vi "Calculate Histogram Data.vi"(7 "Switch X/Y":bool, 11 "Entries":T1[](array[typedef])) -> (3 "Histogram Data":cluster{"X":dbl, "Y":i32}[](array[cluster]))   [LabVIEW 2019, in "Muon Data Post-Processing.lvlib"]
uses:
  Muon Data Post-Processing.lvlib
  <vilib>/Utility/miscctls.llb/LVMapReplaceAction.ctl
  <vilib>/Analysis/NI_AALBase.lvlib
  <vilib>/Analysis/1siggen.llb/Ramp Pattern by Delta.vi
  File Entry.ctl
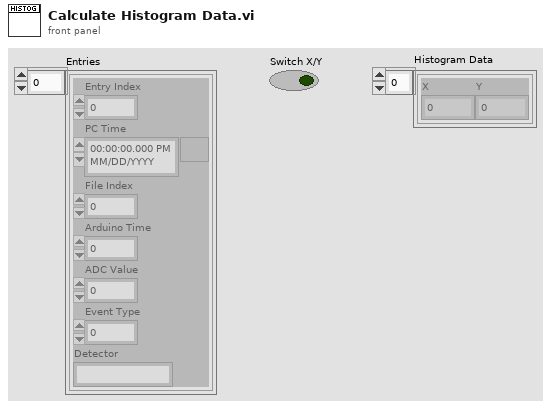
[diagram p1: front panel]
types:
  T1 = typedef "Muon Data Post-Processing.lvlib/File Entry.ctl" = cluster{"Entry Index":i32, "PC Time":timestamp, "File Index":i32, "Arduino Time":i32, "ADC Value":i32, "Event Type":i32, "Detector":string}
  T2 = typedef "LVMapReplaceAction.ctl" = enum32{"Modify Entry only if found", "Add or Modify Entry", "Delete Entry"}
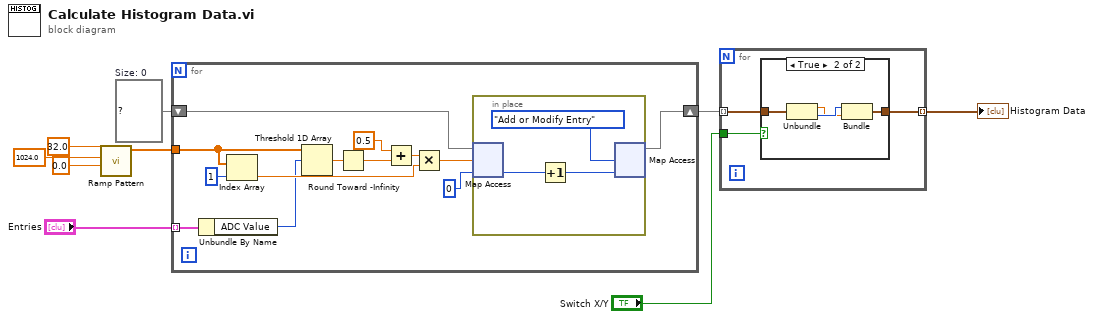
[diagram p0: block diagram]
diagram:
  w4 = map{dbl, i32} {}  # Size: 0
  n1 = call-poly <vilib>:"Ramp Pattern.vi"("start"=0.0, "end"=1024.0, "delta"=32.0) -> ("Ramp Pattern"=w5:dbl[])  [unwired: 6 in, 2 out]
  n2 = for {
    tunnel: "Entries" -> [w22] mode=indexing
    shift-right: [w12] -> w3
    shift-left: w4 -> [w11]
    tunnel: w5 -> [w10]
    n3 = Unbundle By Name(w22) -> ("ADC Value"=w15:i32)
    n4 = Index Array(array=w10, index=1) -> (element=w21:dbl)
    n5 = Threshold 1D Array(2:w15, 3:w10) -> (0:w20:dbl)  [unwired: 1 in]
    n6 = Round Toward -Infinity(1:w20) -> (0:w19:dbl)
    n7 = Add(x=0.5, y=w19) -> (x+y=w18:dbl)
    n8 = Multiply(x=w18, y=w21) -> (x*y=w14:dbl)
    n9 = in-place {
      n10 = in-place-map #1(w11, w14, 0) -> (w25:i32)  [unwired: 1 out]
      n11 = Increment(x=w25) -> (x+1=w24:i32)
      n12 = in-place-map #1(w24, LVMapReplaceAction."Add or Modify Entry" ("action")) -> (w12:map{dbl, i32})  [unwired: 2 out]
    }
  }
  n13 = for {
    tunnel: w3 -> [w27] mode=indexing
    tunnel: [w28] -> w2 mode=indexing
    tunnel: "Switch X/Y" -> [w26]
    n14 = case shown="True" w26 {
      tunnel: [w29 w30] -> w28
      tunnel: w27 -> [w29 w33]
      frame False {
      }
      frame True {
        n15 = Unbundle(w33) -> (w31:dbl, w32:i32)
        n16 = Bundle(w32, w31) -> (w30:cluster{i32, dbl})  [unwired: 1 in]
      }
    }
  }
  "Histogram Data" <- w2
